vi "Page_Dialog_Read.vi"(6 "ctlReferences":T1, 8 "error in (no error)":errorcluster, 11 "Class in":refnum<class "Installer.lvclass">) -> (0 "error out":errorcluster, 3 "Class out":refnum<class "Installer.lvclass">)   [LabVIEW 2020, in "Installer.lvclass"]
uses:
  <vilib>/AppBuilder/IB_Classes/Installer/Installer.lvclass
  <vilib>/AppBuilder/IB_Classes/Installer/Installer.lvclass/Installer.ctl
  <resource>/Framework/Providers/Builds/Installer/CDK_sTypeDef_Languages.ctl
  <resource>/Framework/Providers/Builds/Installer/Pages/controls/IB_UI_Page_Dialog_Info_References.ctl
  <resource>/Framework/Providers/Common/provcom_BrowseProjectFile2.ctl
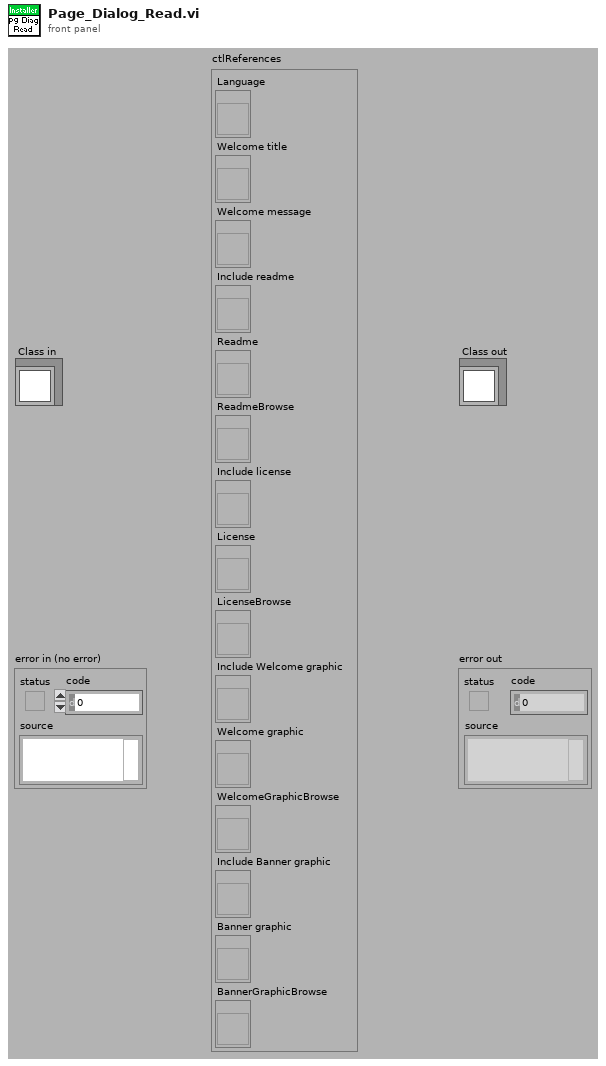
[diagram p1: front panel]
types:
  T1 = typedef "IB_UI_Page_Dialog_Info_References.ctl" = cluster{"Language":refnum<vi>, "Welcome title":refnum<vi>, "Welcome message":refnum<vi>, "Include readme":refnum<vi>, "Readme":refnum<vi>, "ReadmeBrowse":refnum<vi>, "Include license":refnum<vi>, "License":refnum<vi>, "LicenseBrowse":refnum<vi>, "Include Welcome graphic":refnum<vi>, "Welcome graphic":refnum<vi>, "WelcomeGraphicBrowse":refnum<vi>, "Include Banner graphic":refnum<vi>, "Banner graphic":refnum<vi>, "BannerGraphicBrowse":refnum<vi>}
  T2 = typedef "CDK_sTypeDef_Languages.ctl" = u16
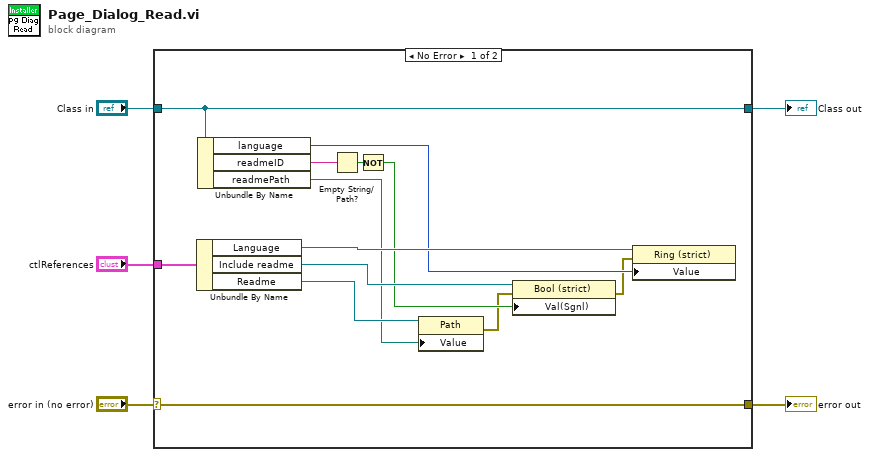
[diagram p0: block diagram]
diagram:
  n1 = case shown="No Error" "error in (no error)" {
    selector: "error in (no error)" -> [w18 w20]
    tunnel: [w18 w20] -> w4
    tunnel: [w17 w19] -> w2
    tunnel: "Class in" -> [w17 w19]
    tunnel: "ctlReferences" -> [w16 _]
    frame No Error {
      n2 = Unbundle By Name(w16) -> ("Language"=w14:refnum<vi>, "Include readme"=w15:refnum<vi>, "Readme"=w9:refnum<vi>)
      n3 = Unbundle By Name(w17) -> ("language"=w13:T2, "readmeID"=w12:string, "readmePath"=w8:path)
      n4 = Empty String/Path?(string/path=w12) -> (empty?=w11:bool)
      n5 = Not(x=w11) -> (.not. x?=w10:bool)
      n6 = property class="Path"(reference=w9, "Value"=w8) -> (error out=w7:errorcluster)  [unwired: 1 in, 1 out]
      n7 = property class="Bool (strict)"(reference=w15, error in=w7, "Val(Sgnl)"=w10) -> (error out=w6:errorcluster)  [unwired: 1 out]
      n8 = property class="Ring (strict)"(reference=w14, error in=w6, "Value"=w13) -> ()  [unwired: 2 out]
    }
    frame Error {
    }
  }
  "error out" <- w4
  "Class out" <- w2
